vi "Build exc Msg.vi"(8 "error in (no error)":errorcluster, 10 "PreT":string, 11 "CurrT":string) -> (0 "error out":errorcluster, 2 "PreMode":string, 3 "CurrMode":string)   [LabVIEW 2014]
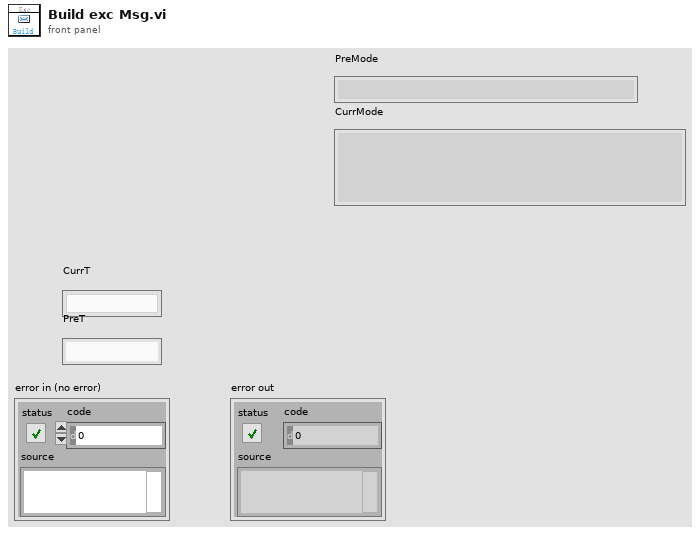
[diagram p1: front panel]
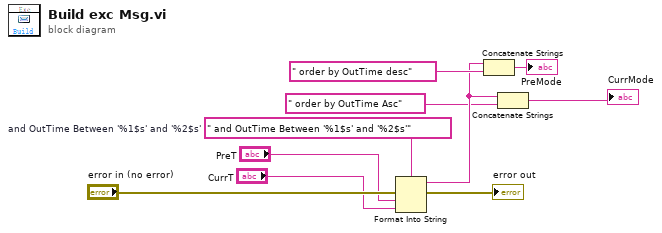
[diagram p0: block diagram]
diagram:
  w9 = " and OutTime Between '%1$s' and '%2$s'"  # and OutTime Between '%1$s' and '%2$s'
  n1 = Format Into String(format string=w9, error in="error in (no error)", "PreT", "CurrT") -> (resulting string=w3:string, error out=→"error out":errorcluster)  [unwired: 1 in]
  n2 = Concatenate Strings(w3, " order by OutTime desc") -> (→"PreMode":string)
  n3 = Concatenate Strings(w3, " order by OutTime Asc") -> (→"CurrMode":string)
